vi "Signel relay command set.vi"(10 "Relay No":i32, 11 "ON/OFF":bool) -> (3 "Command":string)   [LabVIEW 2023, in "Numato.lvlib"]
uses:
  Numato.lvlib
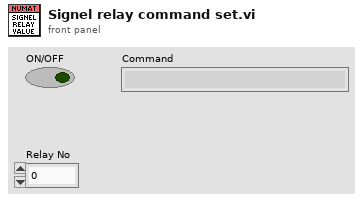
[diagram p1: front panel]
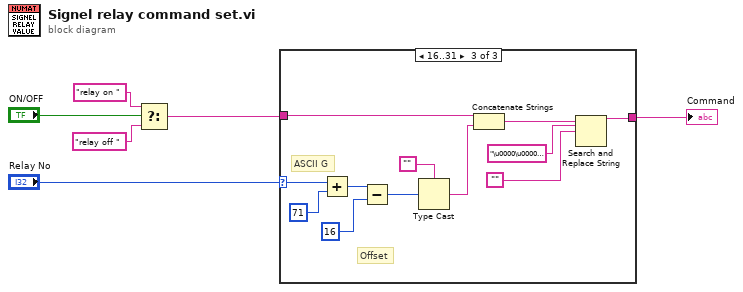
[diagram p0: block diagram]
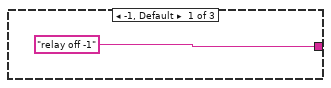
[diagram p2: hidden frame]
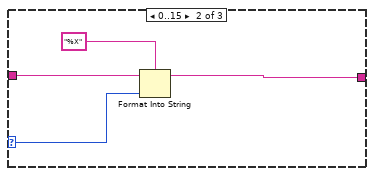
[diagram p3: hidden frame]
diagram:
  n1 = Select(t="relay on ", s="ON/OFF", f="relay off ") -> (s? t:f=w5:string)
  n2 = case shown="16..31" "Relay No" {
    selector: "Relay No" -> [_ w8 w23]
    tunnel: ["relay off -1" w11 w14] -> w6
    tunnel: w5 -> [_ w10 w18]
    frame -1, Default {
    }
    frame 0..15 {
      n3 = Format Into String(format string="%X", initial string=w10, w8) -> (resulting string=w11:string)  [unwired: 1 in, 1 out]
    }
    frame 16..31 {
      # "Offset"
      # "ASCII G"
      n4 = Add(x=w23, y=71) -> (x+y=w21:i32)
      n5 = Subtract(x=w21, y=16) -> (x-y=w19:i32)
      n6 = Type Cast(type="", x=w19) -> (*(type *) &x=w17:string)
      n7 = Concatenate Strings(w18, w17) -> (w15:string)
      n8 = Search and Replace String(input string=w15, search string="\u0000\u0000\u0000" ("Command"), replace string="") -> (result string=w14:string)  [unwired: 5 in, 3 out]
    }
  }
  "Command" <- w6
